vi "onProcessStopped.vi"(8 "error in (no error)":errorcluster, 11 "SMO":refnum<class "SMO.lvclass">) -> (0 "error out":errorcluster, 3 "SMO out":refnum<class "SMO.lvclass">)   [LabVIEW 2013, in "SMO.lvclass"]
uses:
  SMO.lvclass
panel:
  # "For instructions on how to use the JKI State Machine Objects, examples and video tutorials, visit:\nhttp://jki.net/state-machine-objects/\n\nJKI State Machine Objects™\nhttp://jki.net/state-machine-objects/\nCopyright (C) 2005-2015, JKI <info@jki.net>\nALL RIGHTS RESERVED"
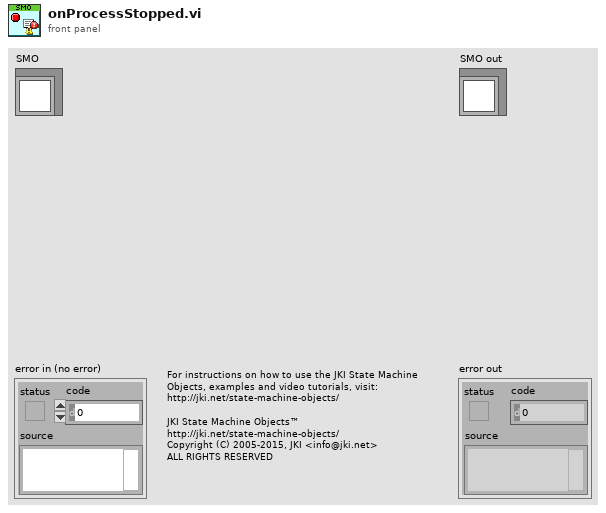
[diagram p1: front panel]
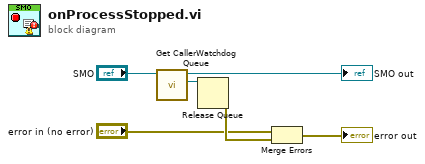
[diagram p0: block diagram]
diagram:
  n1 = call "Get CallerWatchdog Queue.vi"("SMO in"="SMO") -> ("Caller Watchdog"=w6:refnum<queue>, "SMO out"=→"SMO out":refnum<class "SMO.lvclass">)  [unwired: 8 in, 1 out]
  n2 = Release Queue(queue=w6) -> (error out=w3:errorcluster)  [unwired: 2 in, 2 out]
  n3 = Merge Errors("error in (no error)", w3) -> (→"error out":errorcluster)
